vi "CreneauGeneration.vi"() -> (0 "waveform":dbl[](array[numeric]), 3 "Rep Frequency (Hz)":dbl)   [LabVIEW 2016]
uses:
  <vilib>/imath/engines/lvmath2/RunTimeEngine/BuiltInFunctions/nextpowerof2/NIMS_nextpowerof2(GS).vi
  <instcachedir>/0/NIMS_nextpowerof2(GS)_B42BF357393E46BBAF4FDD53A40AE50C.lvgen/NIMS_nextpowerof2(GS)_B42BF357393E46BBAF4FDD53A40AE50C_000.vi
  <vilib>/imath/engines/lvmath2/RunTimeEngine/RangeToken/NIMS_Range.vi
  <instcachedir>/0/NIMS_Range_B290C9A4B417448F8AD7612DC5651788.lvgen/NIMS_Range_B290C9A4B417448F8AD7612DC5651788_000.vi
  <vilib>/imathl/engines/lvmath/Functions/Error Handling/Create Error.vi
  <vilib>/imath/engines/lvmath2/RunTimeEngine/VariableToken/Support/NIMS_Vector Boolean Index to I32 Index.vi
  <vilib>/imath/engines/lvmath2/RunTimeEngine/IndexReplace/NIMS V(V)=S.vi
  <instcachedir>/0/NIMS V(V)=S_C323C74337CB465599A72FED33BE1EA6.lvgen/NIMS V(V)=S_C323C74337CB465599A72FED33BE1EA6_000.vi
  <vilib>/imath/engines/lvmath2/RunTimeEngine/NodeEndStatement/NIMS_NodeEndStatement_Output.vi
  <instcachedir>/0/NIMS_NodeEndStatement_Output_53EC0D466D134D7ABD903AC30B43404B.lvgen/NIMS_NodeEndStatement_Output_53EC0D466D134D7ABD903AC30B43404B_001.vi
  <instcachedir>/0/NIMS_NodeEndStatement_Output_53EC0D466D134D7ABD903AC30B43404B.lvgen/NIMS_NodeEndStatement_Output_53EC0D466D134D7ABD903AC30B43404B_005.vi
  <vilib>/imath/engines/lvmath2/RunTimeEngine/ErrorHandling/NIMS_Finalize Error.vi
panel:
  out "dt":dbl
  in  "Rep Freq (Hz)":dbl
  in  "Tau (us)":dbl=1.0
  in  "Number of data points":u32=131072 min=2 max=131072 step=1
  out "XY Graph 2":cluster{dbl[], "waveform":dbl[]}(graph)
  out "Effective N value (nexpow2)":u32=131072
  in  "OK Button":bool
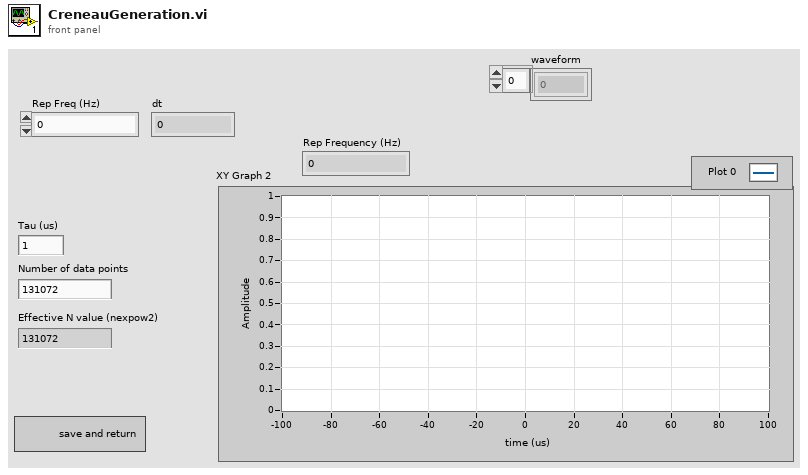
[diagram p1: front panel]
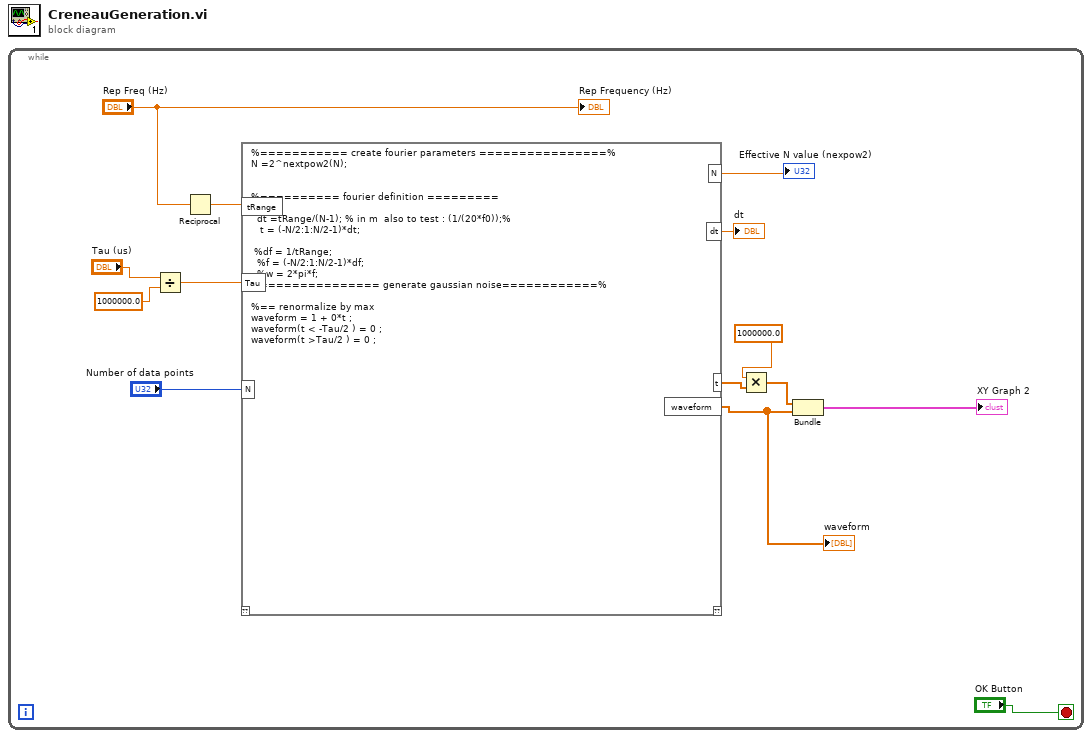
[diagram p0: block diagram]
diagram:
  n1 = while {
    stop <- "OK Button" stop-if-true
    n2 = Divide(x="Tau (us)", y=1000000.0) -> (x/y=w1:dbl)
    n3 = Reciprocal(x="Rep Freq (Hz)") -> (1/x=w4:dbl)
    n4 = mathscript code="%=========== create fourier parameters ================%\nN =2^nextpow2(N);\n\n\n%========== fourier definition =========\n\n  dt =tRange/(N-1); % in m  also to test : (1/(20*f0));%\n   t = (-N/2:1:N/2-1)*dt;\n\n %df = 1/tRange;\n  %f = (-N/2:1:N/2-1)*df;\n  %w = 2*pi*f;\n%=============== generate gaussian noise============%\n\n%== renormalize by max\nwaveform = 1 + 0*t ;\nwaveform(t < -Tau/2 ) = 0 ;\nwaveform(t >Tau/2 ) = 0 ;"("Tau"=w1, "N"="Number of data points", "tRange"=w4) -> ("t"=w7:dbl[], "waveform"=w13:dbl[], "N"=→"Effective N value (nexpow2)":dbl, "dt"=→"dt":dbl)  [unwired: 1 in, 1 out]
    "waveform" <- w13
    n5 = Multiply(x=1000000.0, y=w7) -> (x*y=w5:dbl[])
    n6 = Bundle(w5, "waveform"=w13) -> (→"XY Graph 2":cluster{dbl[], "waveform":dbl[]})  [unwired: 1 in]
    "Rep Frequency (Hz)" <- "Rep Freq (Hz)"
  }
